vi "启动命令国标转换.vi"(11 "启动命令":T2 caption="00：00" items=["", "水样测试", "标样核查", "零点核查", "跨度核查", "空白测试", "平行样测试", "加标回收", "空白校准", "标样校准"]) -> (3 "控制命令":T1)   [LabVIEW 2016, in "定时设置.xctl"]
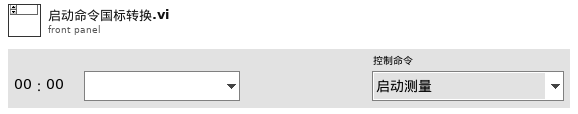
[diagram p1: front panel]
types:
  T1 = typedef "定时设置.xctl/国标控制命令.ctl" = enum16{"启动测量", "标样核查", "零点核查", "跨度核查", "空白测试", "平行样测试", "加标回收", "空白校准", "标样校准", "初始化（清洗）", "停止测试", "仪器重启", "校时", "模式设置", "测量间隔设置"}
  T2 = typedef "定时设置.xctl/启动命令选择.ctl" = u16
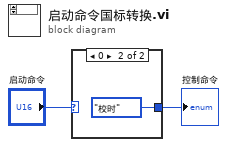
[diagram p0: block diagram]
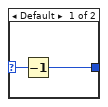
[diagram p2: hidden frame]
diagram:
  n1 = case shown="0" "启动命令" {
    selector: "启动命令" -> [w4 _]
    tunnel: [w3 国标控制命令."校时" ("控制命令")] -> w1
    frame Default {
      n2 = Decrement(x=w4) -> (x-1=w3:T2)
    }
    frame 0 {
    }
  }
  "控制命令" <- w1
